vi "VectorNav Test.vi"() -> ()   [LabVIEW 2010]
uses:
  1.0-Hindbrain Global.vi
panel:
  in  "stop":bool
  in  "VectorNav-Query":bool
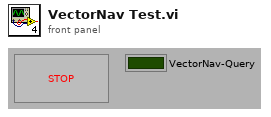
[diagram p1: front panel]
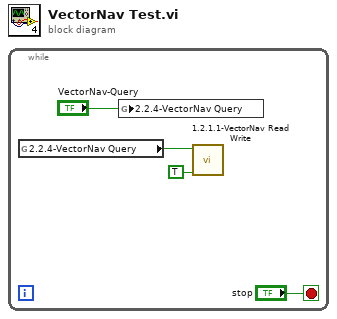
[diagram p0: block diagram]
diagram:
  n1 = while {
    stop <- "stop" stop-if-true
    n2 = global read "1.0-Hindbrain Global.vi" "2.2.4-VectorNav Query"() -> (w2:bool)
    n3 = global write "1.0-Hindbrain Global.vi" "2.2.4-VectorNav Query"("VectorNav-Query") -> ()
    n4 = call "1.2.1.1-VectorNav Read Write.vi"("Stop"=TRUE, "Start"=w2) -> ()  [unwired: 10 in]
  }
